vi "Edit Type Specialization.vi"(11 "error in (no error)":errorcluster) -> (15 "error out":errorcluster)   [LabVIEW 2021, in "Converter.lvlib"]
uses:
  Converter.lvlib
  Path Functions/Path Functions.lvlib
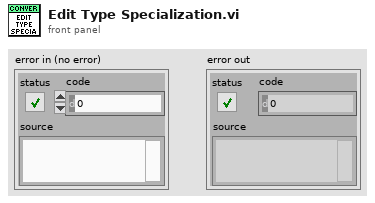
[diagram p1: front panel]
types:
  T1 = cluster{"parameter name":string, "type specialization":enum16{"none", "pin", "path", "enum"}, "annotations":cluster{"key":enum16{"none", "pin.instrument_type", "enum.values"}, "value":string}[]}[]
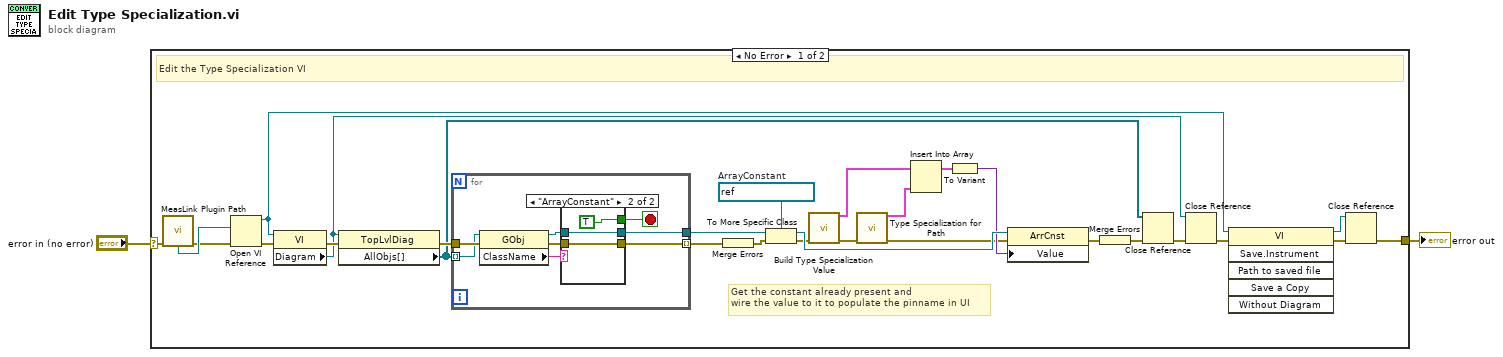
[diagram p0: block diagram]
diagram:
  n1 = case shown="No Error" "error in (no error)" {
    selector: "error in (no error)" -> [w30 w43]
    tunnel: [w19 w43] -> w1
    frame No Error {
      w17 = refnum<vi> refnum  # ArrayConstant
      # "Get the constant already present and\nwire the value to it to populate the pinname in UI"
      # "Edit the Type Specialization VI"
      n2 = call "MeasLink Plugin Path.vi"("error in (no error)"=w30) -> ("Type Specialization"=w29:path, "error out"=w28:errorcluster)  [unwired: 2 in, 11 out]
      n3 = Open VI Reference(vi path=w29, error in (no error)=w28) -> (vi reference=w13:refnum<vi>, error out=w27:errorcluster)  [unwired: 4 in]
      n4 = property class="VI"(reference=w13, error in=w27) -> (error out=w26:errorcluster, "Diagram"=w20:refnum<vi>)  [unwired: 1 out]
      n5 = property class="TopLvlDiag"(reference=w20, error in=w26) -> (error out=w25:errorcluster, "AllObjs[]"=w21:refnum<vi>[])  [unwired: 1 out]
      n6 = for {
        tunnel: w21 -> [w37] mode=indexing
        tunnel: w25 -> [w38]
        tunnel: [w33] -> w18
        tunnel: [w31] -> w16 mode=indexing
        stop <- w32 stop-if-true
        n7 = property class="GObj"(reference=w37, error in=w38) -> (reference out=w34:refnum<vi>, error out=w35:errorcluster, "ClassName"=w36:string)
        n8 = case shown="\"ArrayConstant\"" w36 {
          tunnel: w35 -> [w39 w40]
          tunnel: w34 -> [_ w42]
          tunnel: [_ w42] -> w33
          tunnel: [_ TRUE] -> w32
          tunnel: [w39 w40] -> w31
          frame Default {
          }
          frame "ArrayConstant" {
          }
        }
      }
      n9 = Merge Errors(w16) -> (w15:errorcluster)
      n10 = To More Specific Class(target class=w17, reference=w18, error in=w15) -> (specific class reference=w12:refnum<vi>, error out=w11:errorcluster)
      n11 = call "Build Type Specialization Value.vi"("error in (no error)"=w11) -> ("Type Specialization"=w7:T1, "error out"=w5:errorcluster)  [unwired: 13 in]
      n12 = call "Type Specialization for Path.vi"("error in (no error)"=w5) -> ("Type Specialization for Path"=w6:T1, "error out"=w4:errorcluster)  [unwired: 13 in]
      n13 = Insert Into Array(array=w7, new element=w6) -> (w3:T1)  [unwired: 1 in]
      n14 = To Variant(anything=w3) -> (Variant=w10:variant)
      n15 = property class="ArrCnst"(reference=w12, error in=w4, "Value"=w10) -> (error out=w9:errorcluster)  [unwired: 1 out]
      n16 = Merge Errors(w9) -> (w24:errorcluster)
      n17 = Close Reference(reference=w21, error in (no error)=w24) -> (error out=w23:errorcluster)
      n18 = Close Reference(reference=w20, error in (no error)=w23) -> (error out=w22:errorcluster)
      n19 = invoke class="VI" method="Save.Instrument"(reference=w13, error in=w22) -> (reference out=w8:refnum<vi>, error out=w14:errorcluster)  [unwired: 4 in, 4 out]
      n20 = Close Reference(reference=w8, error in (no error)=w14) -> (error out=w19:errorcluster)
    }
    frame Error {
    }
  }
  "error out" <- w1
